vi "RangeSearch.vi"() -> ()   [LabVIEW 2019]
panel:
  in  "stop":bool
  out "Array 2 Value":dbl
  out "Array 1 Value":dbl
  out "Array Index":dbl
  out "Search Value":dbl
  in  "Search Value":dbl(slide) scale=9.0..14.0
  out "Fractional Index":dbl
  out "Searched Part of 2D Array":dbl[](array[numeric])
  out "Input File":string
  out "Output Array":dbl[][](array[numeric])
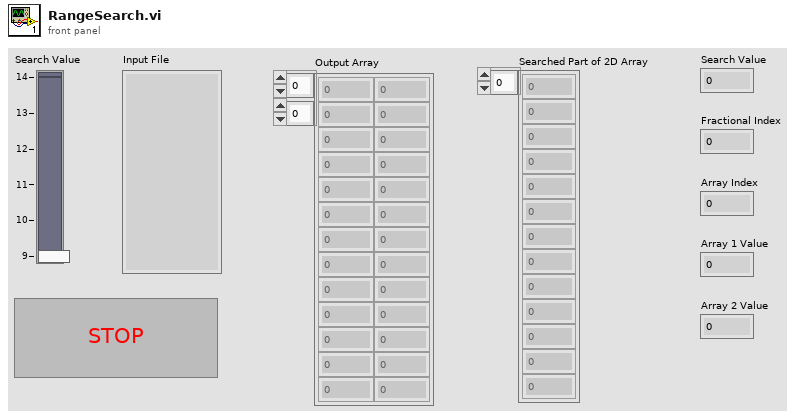
[diagram p1: front panel]
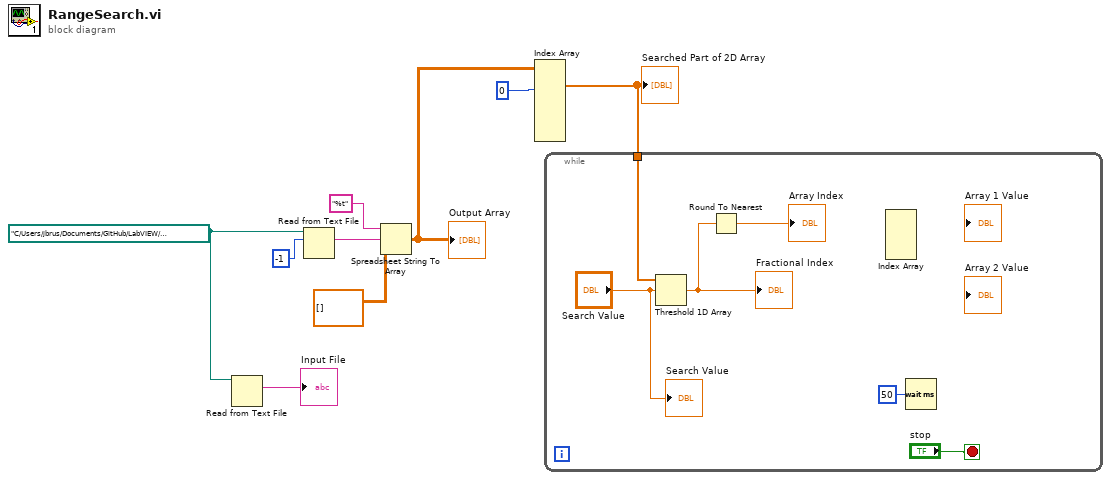
[diagram p0: block diagram]
diagram:
  w6 = path "C:/Users/jbrus/Documents/GitHub/LabVIEW/3LabVIEW-Specific-Features/FileInput/InputFile2.txt"
  n1 = Read from Text File(file (use dialog)=w6) -> (text=→"Input File":string)  [unwired: 3 in, 3 out]
  n2 = Read from Text File(file (use dialog)=w6, count=-1) -> (text=w9:string)  [unwired: 2 in, 3 out]
  n3 = Spreadsheet String To Array(format string="%t", spreadsheet string=w9, array type (2D Dbl)=dbl[][] []) -> (array=w3:dbl[][])  [unwired: 1 in]
  "Output Array" <- w3
  n4 = Index Array(array=w3, index (col) #1=0 ("disabled index (col)")) -> (element #1=w1:dbl[])  [unwired: 7 in, 3 out]
  "Searched Part of 2D Array" <- w1
  n5 = while {
    tunnel: w1 -> [w15]
    stop <- "stop" stop-if-true
    n6 = Threshold 1D Array(2:"Search Value", 3:w15) -> (0:w10:dbl)  [unwired: 1 in]
    "Fractional Index" <- w10
    n7 = Round To Nearest(number=w10) -> (nearest integer value=→"Array Index":dbl)
    n8 = Index Array() -> ()  [unwired: 5 in, 4 out]
    n9 = Wait (ms)(milliseconds to wait=u32 50) -> ()  [unwired: 1 out]
    "Search Value" <- "Search Value"
  }
